vi "RemoveShotsFromArray.vi"(8 "IntensityArray_IN":u8[][](array[numeric]), 10 "Indexes":i32[](array[numeric]), 11 "ShotArray_IN":T1[](array[typedef])) -> (0 "IntensityArray_OUT":u8[][](array[numeric]), 3 "ShotArray_OUT":T1[](array[typedef]))   [LabVIEW 2022 SP3]
uses:
  ShotCluster.ctl
  move_dir_ud.ctl
  98d2586a-a126-421e-9760-2507514c154c.vi
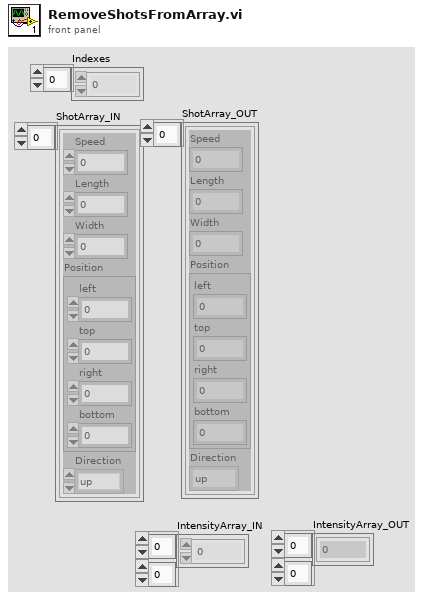
[diagram p1: front panel]
types:
  T1 = typedef "ShotCluster.ctl" = cluster{"Speed":u32, "Length":u32, "Width":u32, "Position":cluster{"left":i16, "top":i16, "right":i16, "bottom":i16}, "Direction":T2}
  T2 = typedef "move_dir_ud.ctl" = enum16{"up", "down"}
  T3 = cluster{"left":i16, "top":i16, "right":i16, "bottom":i16}
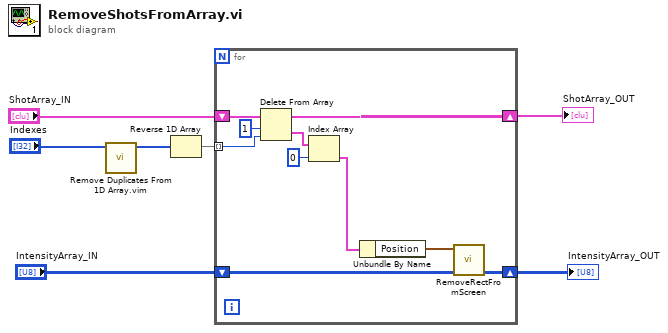
[diagram p0: block diagram]
diagram:
  n1 = call "Remove Duplicates From 1D Array.vim"("array"="Indexes") -> ("array with duplicates removed"=w6:i32[])  [unwired: 10 in]
  n2 = Reverse 1D Array(array=w6) -> (reversed array=w4:i32[])
  n3 = for {
    shift-right: [w16] -> w3
    shift-left: "ShotArray_IN" -> [w17]
    tunnel: w4 -> [w14] mode=indexing
    shift-right: [w10] -> w1
    shift-left: "IntensityArray_IN" -> [w11]
    n4 = Delete From Array(array=w17, length=1, index=w14) -> (deleted portion=w13:T1[], array with subset deleted=w16:T1[])
    n5 = Index Array(array=w13, index=0) -> (element=w9:T1)
    n6 = Unbundle By Name(w9) -> ("Position"=w8:T3)
    n7 = call "RemoveRectFromScreen.vi"("IntensityArray_IN"=w11, "Position"=w8) -> ("IntensityArray_OUT"=w10:u8[][])  [unwired: 9 in]
  }
  "ShotArray_OUT" <- w3
  "IntensityArray_OUT" <- w1
